vi "PointMassSimulation.vi"() -> ()   [LabVIEW 2016]
uses:
  <vilib>/addons/Control Design/_Model Construction/Model Typedefs.llb/CD State Space Model (MIMO).ctl
  <vilib>/addons/Control Design/_Model Construction/Model Typedefs.llb/CD General Elements.ctl
  <vilib>/Platform/TimedLoop/XDataNode/timing_clust.ctl
  <vilib>/Platform/TimedLoop/XDataNode/nitl_modes.ctl
  <vilib>/Platform/TimedLoop/XDataNode/wakeup.ctl
  <vilib>/Simulation/DiscreteLinear/Implementation/NILVSim Discrete State Space Direct.llb/SIM Discrete State Space Direct Diagram (CD).vi
  <vilib>/Simulation/DiscreteLinear/Implementation/Shared/SIM Init Discrete States.vi
  <vilib>/Simulation/DiscreteLinear/Implementation/NILVSim Discrete State Space Direct.llb/NILVSim Discrete State Space Direct Diagram Core (MIMO).vi
  <vilib>/FPGAPlugInAG/roboRIO/niLvFpga_Open_roboRIO.vi
  <vilib>/rvi/interface/common/dynamic/niFpgaDynamicAddResources.vi
  <vilib>/FPGAPlugInAG/Dynamic/niLvFpga_Reset_Dynamic.vi
  <vilib>/imath/engines/lvmath2/RunTimeEngine/Managers/WorkSpace/UID Generator.vi
  <vilib>/imath/engines/lvmath/Plug In/Control Design/BuiltInFunctions/ss/NIMS_CD_ss(A,B,C,D).vi
  <vilib>/imath/engines/lvmath/Plug In/Control Design/BuiltInFunctions/c_to_d/NIMS_CD_c_to_d(SS,TS,STR,DBL).vi
  <vilib>/imath/engines/lvmath2/RunTimeEngine/RunTimeType/NIMS_RunTimeType_From StrictType (excl LVString).vi
  <instcachedir>/0/NIMS_RunTimeType_From StrictType (excl LVString)_BBF44FB49F834B71AF7A14CCEDF8BECD.lvgen/NIMS_RunTimeType_From StrictType (excl LVString)_BBF44FB49F834B71AF7A14CCEDF8BECD_031.vi
  <vilib>/imath/engines/lvmath2/RunTimeEngine/LocalVariableDefStatement/MC_LocalVariableDefStatement_Display.vi
  <vilib>/imath/engines/lvmath2/RunTimeEngine/Managers/SymbolTable/Clear UID.vi
  <vilib>/imath/engines/lvmath2/RunTimeEngine/NodeEndStatement/NIMS_NodeEndStatement_Output.vi
  <instcachedir>/0/NIMS_NodeEndStatement_Output_53EC0D466D134D7ABD903AC30B43404B.lvgen/NIMS_NodeEndStatement_Output_53EC0D466D134D7ABD903AC30B43404B_001.vi
  <instcachedir>/0/NIMS_NodeEndStatement_Output_53EC0D466D134D7ABD903AC30B43404B.lvgen/NIMS_NodeEndStatement_Output_53EC0D466D134D7ABD903AC30B43404B_010.vi
  <vilib>/imath/engines/lvmath2/RunTimeEngine/ErrorHandling/NIMS_Finalize Error.vi
  <vilib>/FPGAPlugInAG/Dynamic/niLvFpga_Run_Dynamic.vi
  <vilib>/Utility/error.llb/Error Cluster From Error Code.vi
  <vilib>/rvi/errors/niLvFpgaAdjustHostInterfaceError.vi
  <vilib>/addons/control/pid/pid.llb/PID (DBL).vi
  <vilib>/FPGAPlugInAG/Dynamic/niLvFpga_Close_Dynamic.vi
  <vilib>/Simulation/Implementation/Shared/SIM BuildSimErr.vi
  <vilib>/rvi/interface/nirviOpenFPGA/nirviOpenFPGA.xnode
  FPGA Bitfiles/AutoBikeProject_FPGATarget_SteeringControlS_sPMkvCApzNQ.lvbitx
  <vilib>/rvi/interface/nirviMethod/nirviMethod.xnode
  <vilib>/rvi/interface/nirviReadWriteControl/nirviReadWriteControl.xnode
  <vilib>/rvi/interface/nirviCloseFPGA/nirviCloseFPGA.xnode
  <vilib>/Platform/TimedLoop/XDataNode/XDataNode.xnode
  <vilib>/Simulation/Implementation/XNodeFramework/SimXNode/SimX.xnode
  <vilib>/addons/control/pid/NI_PID_pid.lvlib
  <vilib>/rvi/interface/Simulation/niFpgaSimulationCallBeginRW.vi
  <vilib>/Platform/TimedLoop/XDataNode/XDNodeRunTimeDep.lvlib
  <vilib>/addons/Control Design/_Model Construction/NI_LinSys_Model Typedefs.lvlib
  NiFpgaLv.dll
  <vilib>/imath/engines/lvmath2/RunTimeEngine/Managers/SymbolTable/NIMS_WorkSpace.lvlib
  <vilib>/addons/control/pid/NI_PID_autopid.lvlib
panel:
  in  "initial state (x0)":dbl[](array[numeric])=[0.0]
  out "PID gains out":T1={"proportional gain (Kc)"=1.0, "integral time (Ti, min)"=0.01, "derivative time (Td, min)"=0.0} {"derivative time (Td, min)" format="%.3f"; "integral time (Ti, min)" format="%.3f"; "proportional gain (Kc)" format="%.3f"}
  out "tuning completed?":bool
  in  "reinitialize? (F)":bool
  in  "Autotuning?":bool
  in  "v_in":dbl format="%#_13g"
  out "accual PID values 2":T2
  out "Desired steer":sgl
  out "Steering loop time":u32
  in  "Loop itr":i32=2
  out "Duty cycle":dbl
  out "error out":errorcluster
  out "stop":bool
  out "Finished Late? [i-1]":bool
  out "Steering":dbl
  out "Lean":dbl
  in  "setpoint weighting":T3
  in  "output range":T4
  in  "gains":T5
  in  "error in":errorcluster
  out "Lean angle":dbl(graph)
  out "Steer angle":dbl(graph)
  in  "Balancing gains":T1={"proportional gain (Kc)"=1.0, "integral time (Ti, min)"=0.01, "derivative time (Td, min)"=0.0} {"derivative time (Td, min)" format="%.3f"; "integral time (Ti, min)" format="%.3f"; "proportional gain (Kc)" format="%.3f"}
  out "sys":T6 caption="SS object" {"Transport Delay" format="%.2f"; "D" format="%#.2g"; "C" format="%#.2g"; "B" format="%#.2g"; "A" format="%#.2g"; "properties"."Sampling Time" format="%#.6p"; "properties"."Output Delays" format="%.4f"; "properties"."Input Delays" format="%.4f"}
  # "lean"
  # "lean velocity"
  # "steer"
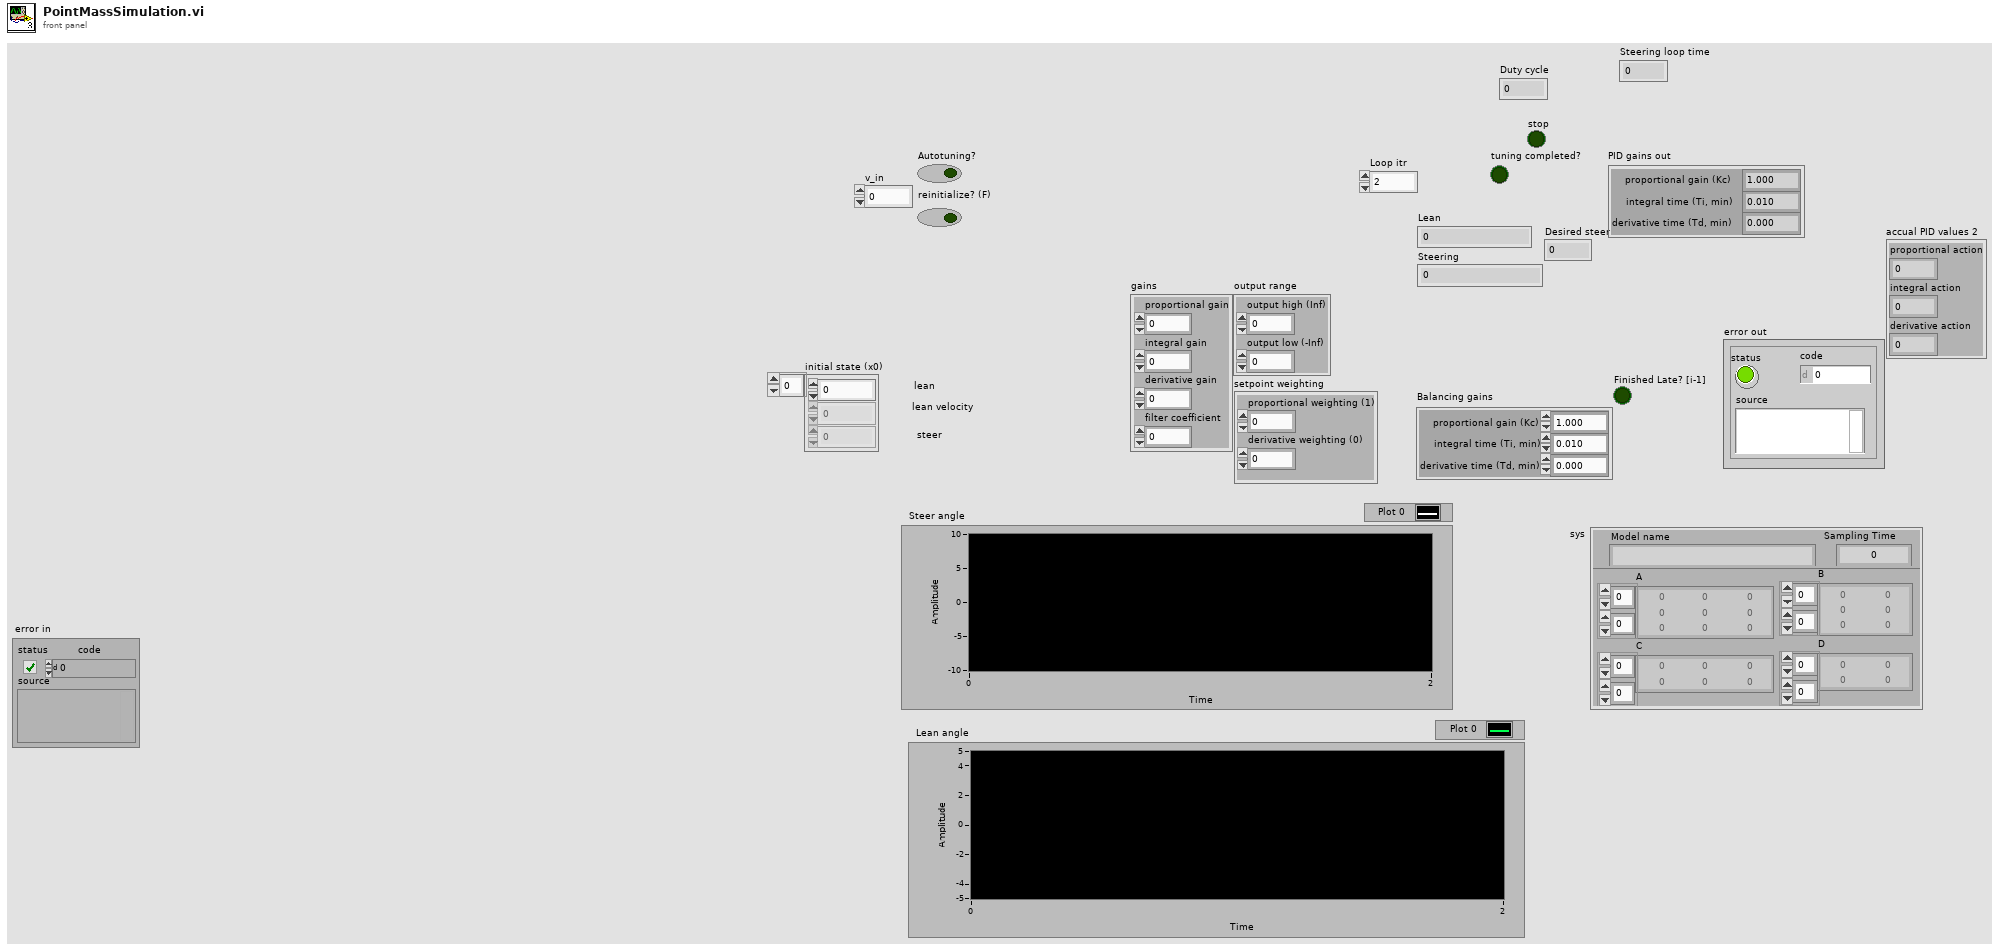
[diagram p1: front panel]
types:
  T1 = cluster{"proportional gain (Kc)":dbl, "integral time (Ti, min)":dbl, "derivative time (Td, min)":dbl}
  T2 = cluster{"proportional action":sgl, "integral action":sgl, "derivative action":sgl}
  T3 = cluster{"proportional weighting (1)":sgl, "derivative weighting (0)":sgl}
  T4 = cluster{"output high (Inf)":sgl, "output low (-Inf)":sgl}
  T5 = cluster{"proportional gain":sgl, "integral gain":sgl, "derivative gain":sgl, "filter coefficient":sgl}
  T6 = typedef "NI_LinSys_Model Typedefs.lvlib/CD State Space Model (MIMO).ctl" = cluster{"properties":T7, "A":dbl[][], "B":dbl[][], "C":dbl[][], "D":dbl[][], "StateNames":string[], "Transport Delay":dbl[][]}
  T7 = typedef "NI_LinSys_Model Typedefs.lvlib/CD General Elements.ctl" = cluster{"Model name":string, "Input names":string[], "Output names":string[], "Input Delays":dbl[], "Output Delays":dbl[], "Sampling Time":dbl, "Notes":string}
  T8 = typedef "XDNodeRunTimeDep.lvlib/timing_clust.ctl" = cluster{"Expected End [f-1]":u64, "Actual End [f-1]":u64, "Finished Late? [f-1]":bool, "Expected End [i-1]":u64, "Actual End [i-1]":u64, "Finished Late? [i-1]":bool, "Expected Start [i]":u64, "Actual Start [i]":u64, "Expected Start [f]":u64, "Actual Start [f]":u64, "Source Name":string, "Structure Name":string, "Period":i64, "Deadline":i64, "Offset":i64, "Start":i64, "Priority":i32, "Timeout":i32, "Mode":T9, "Wakeup Reason":T10, "Error":errorcluster, "Source Type":string, "Secondary Source Type":string, "Global End Time":u64, "Global Start Time":u64, "Frame Duration":u64, "Iteration Duration":u64, "Assigned CPU":i32, "I/O Scan Engine Mode":u32}
  T9 = typedef "XDNodeRunTimeDep.lvlib/nitl_modes.ctl" = enum32{"No Change", "Process missed periods, maintain original phase", "Discard missed periods, maintain original phase", "Process missed periods, ignore original phase", "Discard missed periods, ignore original phase"}
  T10 = typedef "XDNodeRunTimeDep.lvlib/wakeup.ctl" = enum32{"Normal", "Aborted", "Asynchronous wakeup", "Timing source error", "Timed loop error", "Timeout"}
  T11 = cluster{"controller type":u16, "relay cycles":i32, "relay amplitude":dbl, "control specification":u16, "PV noise level":dbl}
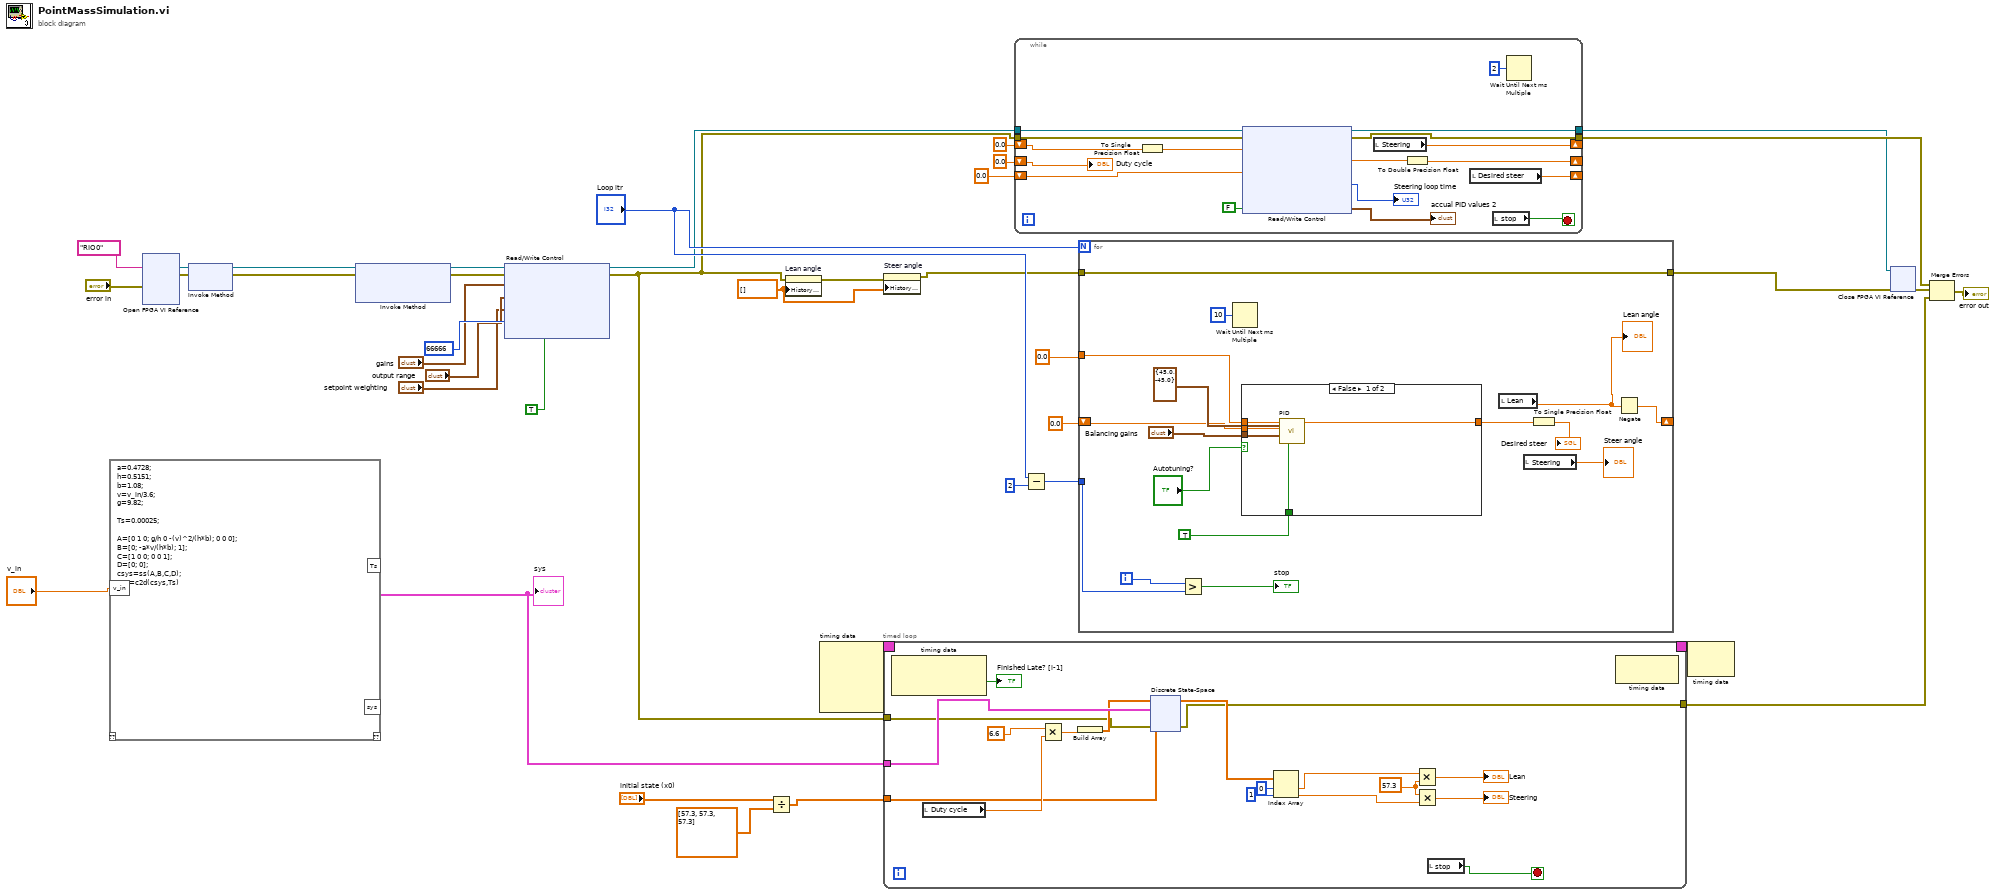
[diagram p0: block diagram]
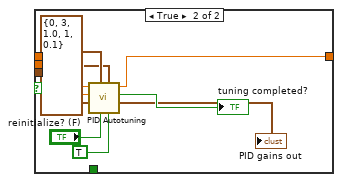
[diagram p2: hidden frame]
diagram:
  w5 = dbl[] [] ("History Data")
  n1 = mathscript code="a=0.4728;\nh=0.5151;\nb=1.08;\nv=v_in/3.6;\ng=9.82;\n\nTs=0.00025;\n\nA=[0 1 0; g/h 0 -(v)^2/(h*b); 0 0 0];\nB=[0; -a*v/(h*b); 1];\nC=[1 0 0; 0 0 1];\nD=[0; 0];\ncsys=ss(A,B,C,D);\nsys=c2d(csys,Ts)"("v_in"="v_in") -> ("sys"=w29:T6)  [unwired: 1 in, 2 out]
  "sys" <- w29
  n2 = xnode "Open FPGA VI Reference"("error in"="error in", "resource name"=tag "RIO0") -> ("FPGA VI Reference Out"=w38:refnum<k20>, "error out"=w39:errorcluster)
  n3 = xnode "Invoke Method"("FPGA VI Reference In"=w38, "error in"=w39) -> ("FPGA VI Reference Out"=w34:refnum<k20>, "error out"=w33:errorcluster)
  n4 = xnode "Invoke Method"("FPGA VI Reference In"=w34, "error in"=w33) -> ("FPGA VI Reference Out"=w35:refnum<k20>, "error out"=w36:errorcluster)  [unwired: 1 in]
  n5 = xnode "Read/Write Control"("FPGA VI Reference In"=w35, "error in"=w36, "gains"="gains", "output range"="output range", "setpoint weighting"="setpoint weighting", "loop wait time (ticks)"=u32 66666, "Pid reset (F)"=TRUE) -> ("FPGA VI Reference Out"=w13:refnum<k20>, "error out"=w8:errorcluster)
  n6 = Divide(x="initial state (x0)", y=dbl[] [57.3, 57.3, 57.3]) -> (x/y=w3:dbl[])
  n7 = property on="Lean angle" class="WFChart (strict)"(error in=w8, "History Data"=w5) -> (error out=w7:errorcluster)  [unwired: 1 in, 1 out]
  n8 = node-c288() -> (w31:T8)  [unwired: 4 in]
  n9 = property on="Steer angle" class="WFChart (strict)"(error in=w7, "History Data"=w5) -> (error out=w6:errorcluster)  [unwired: 1 in, 1 out]
  n10 = timed-loop {
    timing: w31 -> [_]
    timing-out: [_] -> w30
    tunnel: w29 -> [w54]
    tunnel: w8 -> [w43]
    tunnel: [w42] -> w25
    tunnel: w3 -> [w40]
    stop <- w55 stop-if-true
    w53 = 57.3 ("y")
    n11 = node-c288() -> (→"Finished Late? [i-1]":bool)  [unwired: 1 in, 1 out]
    n12 = local read "Duty cycle"() -> (w51:dbl)
    n13 = Multiply(x=6.6 ("y 2"), y=w51) -> (x*y=w50:dbl)
    n14 = Build Array(w50) -> (w49:dbl[])
    n15 = xnode ("Discrete State-Space")("input u(k)"=w49, "State-Space"=w54, "initial state (x0)"=w40, "error in (no error)"=w43) -> ("output y(k)"=w48:dbl[], "error out"=w42:errorcluster)  [unwired: 1 in, 2 out]
    n16 = Index Array(array=w48, index #1=0 ("index"), index #2=1 ("index")) -> (element #1=w45:dbl, element #2=w44:dbl)
    n17 = Multiply(x=w45, y=w53) -> (x*y=→"Lean":dbl)
    n18 = Multiply(x=w53, y=w44) -> (x*y=→"Steering":dbl)
    n19 = local read "stop"() -> (w55:bool)
    n20 = node-c288() -> ()  [unwired: 1 in, 1 out]
  }
  n21 = while {
    shift-right: [w85] -> _
    shift-left: 0.0 ("Steering") -> [w84]
    shift-right: [w81] -> _
    shift-left: 0.0 -> [w80]
    shift-right: [w76] -> _
    shift-left: sgl 0.0 ("Desired steer") -> [w75]
    tunnel: w13 -> [w74]
    tunnel: [w73] -> w11
    tunnel: w8 -> [w72]
    tunnel: [w71] -> w12
    stop <- w70 stop-if-true
    n22 = To Single Precision Float(number=w84) -> (single precision float=w83:sgl)
    n23 = xnode "Read/Write Control"("FPGA VI Reference In"=w74, "error in"=w72, "Current steering angle"=w83, "Desired steering angle"=w75, "Pid reset (F)"=FALSE) -> ("FPGA VI Reference Out"=w73:refnum<k20>, "error out"=w71:errorcluster, "Duty cycle (steering)"=w82:sgl, "Steering loop time"=→"Steering loop time":u32, "accual PID values"=→"accual PID values 2":T2)
    n24 = local read "Steering"() -> (w85:dbl)
    n25 = To Double Precision Float(number=w82) -> (double precision float=w81:dbl)
    n26 = local read "Desired steer"() -> (w76:sgl)
    n27 = local read "stop"() -> (w70:bool)
    n28 = Wait Until Next ms Multiple(millisecond multiple=u32 2) -> ()  [unwired: 1 out]
    "Duty cycle" <- w80
  }
  n29 = Subtract(x="Loop itr", y=2) -> (x-y=w21:i32)
  n30 = for {
    N: "Loop itr" -> [_]
    tunnel: w6 -> [w94]
    shift-right: [w91] -> _
    shift-left: 0.0 ("Lean") -> [w96]
    tunnel: [w94] -> w27
    tunnel: w21 -> [w95]
    tunnel: 0.0 ("setpoint") -> [w93]
    i -> [w97]
    n31 = Greater?(x=w97, y=w95) -> (0:→"stop":bool)
    n32 = Wait Until Next ms Multiple(millisecond multiple=u32 10) -> ()  [unwired: 1 out]
    n33 = case shown="False" "Autotuning?" {
      tunnel: [w108 w112] -> w102
      tunnel: cluster{"output high":dbl, "output low":dbl} {"output high"=45.0, "output low"=-45.0} ("output range") -> [w107 w110]
      tunnel: "Balancing gains" -> [w106 w116]
      tunnel: w96 -> [w105 w117]
      tunnel: w93 -> [w104 w118]
      tunnel: TRUE ("reinitialize? (F)") -> [w103 _]
      frame False {
        n34 = call-poly <vilib>:"PID.vi"("reinitialize? (F)"=w103, "output range"=w107, "PID gains"=w106, "process variable"=w105, "setpoint"=w104) -> ("output"=w108:dbl)  [unwired: 5 in, 1 out]
      }
      frame True {
        n35 = call <vilib>:"PID Autotuning.vi"("autotune? (F)"=TRUE, "autotuning parameters"=T11 {"controller type"=0, "relay cycles"=3, "relay amplitude"=1.0, "control specification"=1, "PV noise level"=0.1}, "reinitialize? (F)"="reinitialize? (F)", "output range"=w110, "PID gains"=w116, "process variable"=w117, "setpoint"=w118) -> ("PID gains out"=→"PID gains out":T1, "tuning completed?"=→"tuning completed?":bool, "output"=w112:dbl)  [unwired: 1 in, 1 out]
      }
    }
    n36 = local read "Lean"() -> (w88:dbl)
    "Lean angle" <- w88
    n37 = local read "Steering"() -> (→"Steer angle":dbl)
    n38 = To Single Precision Float(number=w102) -> (single precision float=→"Desired steer":sgl)
    n39 = Negate(x=w88) -> (-x=w91:dbl)
  }
  n40 = node-c288(w30) -> ()  [unwired: 1 out]
  n41 = xnode "Close FPGA VI Reference"("FPGA VI Reference In"=w11, "error in"=w27) -> ("error out"=w26:errorcluster)
  n42 = Merge Errors(w12, w26, w25) -> (→"error out":errorcluster)
